vi "Apply.vi"(8 "error in":errorcluster, 11 "AO DAQmx DC Simulated CFG in":refnum<class "AO DAQmx DC Simulated CFG.lvclass">) -> (0 "error out":errorcluster, 3 "AO DAQmx DC Simulated CFG out":refnum<class "AO DAQmx DC Simulated CFG.lvclass">)   [LabVIEW 2023, in "DAQmx Simulated CFGs.lvlib" / "AO DAQmx DC Simulated CFG.lvclass"]
uses:
  AO DAQmx DC Simulated CFG.lvclass
  AO DAQmx DC Simulated CFG.lvclass/AO DAQmx DC Simulated CFG.ctl
  AO DAQmx DC CFG/AO DAQmx DC CFG.lvclass
  Configuration/Configuration JSON/Configuration JSON Base/CFG JSON.lvclass
  D:/git/HAL/HAL GOOP4/AO/AO DAQmx DC CFG/AO DAQmx DC CFG.lvclass
  D:/git/HAL/HAL GOOP4/DAQmx/DAQmx Base CFG/DAQmx Base CFG.lvclass
  D:/git/HAL/HAL GOOP4/CFG Target/CFG Target.lvclass
  D:/git/HAL/HAL GOOP4/Configuration/Configuration Semaphore/CFG Semaphore.lvclass
  D:/git/HAL/HAL GOOP4/Configuration/Configuration JSON/Configuration JSON Base/CFG JSON.lvclass
  D:/git/HAL/HAL GOOP4/Interfaces/IConfigure/IConfigure.lvclass
  D:/git/HAL/HAL GOOP4/AO/AO DAQmx DC Simulated CFG/AO DAQmx DC Simulated CFG.lvclass
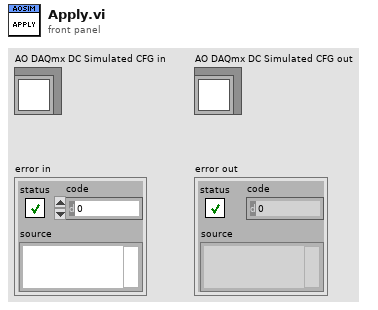
[diagram p1: front panel]
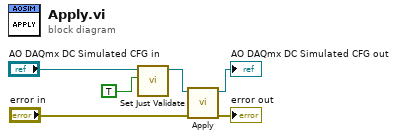
[diagram p0: block diagram]
diagram:
  n1 = call "Set Just Validate.vi"("Just Validate"=TRUE, "CFG JSON Base in"="AO DAQmx DC Simulated CFG in") -> ("CFG JSON Base out"=w2:refnum<class "AO DAQmx DC Simulated CFG.lvclass">)  [unwired: 9 in]
  n2 = call-parent "Apply.vi"("error in"="error in", "AO DAQmx DC CFG in"=w2) -> ("error out"=→"error out":errorcluster, "AO DAQmx DC CFG out"=→"AO DAQmx DC Simulated CFG out":refnum<class "AO DAQmx DC Simulated CFG.lvclass">)  [unwired: 8 in]
